vi "FPGAmain_5782_AM_PID.vi"() -> ()   [LabVIEW 2013]
uses:
  FPGA/DataMode.ctl
  FPGA/Input_5782/5782_states.ctl
  <vilib>/Platform/TimedLoop/XDataNode/timing_clust.ctl
  <vilib>/Platform/TimedLoop/XDataNode/nitl_modes.ctl
  <vilib>/Platform/TimedLoop/XDataNode/wakeup.ctl
  <vilib>/rvi/Emulation/niFpgaSctlEmulationGetInTimedLoop.vi
  <vilib>/rvi/Emulation/niFpgaEmulationReportErrorSimple.vi
  <vilib>/rvi/Emulation/niFpgaGetClockAttributes.vi
  <vilib>/rvi/eio/common/nirviEmuTemplateMethod_errors.vi
  <vilib>/rvi/Emulation/niFpgaCriticalErrorInLSC.vi
  <vilib>/rvi/DataTransferAndStorage/Register/Emulation/niFpgaRegisterEmulationFpgaImpl.vi
  <instcachedir>/0/niFpgaRegisterEmulationFpgaImpl_DCF4BC0110594B98B44A971D60CEEC4D.lvgen/niFpgaRegisterEmulationFpgaImpl_DCF4BC0110594B98B44A971D60CEEC4D_003.vi
  <vilib>/rvi/DataTransferAndStorage/Container/Common/niFpgaContainerGetUniqueNameForEmu.vi
  <instcachedir>/0/niFpgaRegisterEmulationFpgaImpl_DCF4BC0110594B98B44A971D60CEEC4D.lvgen/niFpgaRegisterEmulationFpgaImpl_DCF4BC0110594B98B44A971D60CEEC4D_021.vi
  <instcachedir>/0/niFpgaRegisterEmulationFpgaImpl_DCF4BC0110594B98B44A971D60CEEC4D.lvgen/niFpgaRegisterEmulationFpgaImpl_DCF4BC0110594B98B44A971D60CEEC4D_020.vi
  <instcachedir>/0/niFpgaRegisterEmulationFpgaImpl_DCF4BC0110594B98B44A971D60CEEC4D.lvgen/niFpgaRegisterEmulationFpgaImpl_DCF4BC0110594B98B44A971D60CEEC4D_010.vi
  <instcachedir>/0/niFpgaRegisterEmulationFpgaImpl_DCF4BC0110594B98B44A971D60CEEC4D.lvgen/niFpgaRegisterEmulationFpgaImpl_DCF4BC0110594B98B44A971D60CEEC4D_009.vi
  <vilib>/rvi/FIFO/Fifo_Resource/nirvififoEmulationReadFpgaImpl.vi
  <vilib>/rvi/interface/RandomDataEmulation/nirviRandomDataMultiElementFPGAFIFO.vi
  <instcachedir>/0/nirviRandomDataMultiElementFPGAFIFO_F2B80EDE0D7944A08478D8D26097D4DB.lvgen/nirviRandomDataMultiElementFPGAFIFO_F2B80EDE0D7944A08478D8D26097D4DB_005.vi
  <vilib>/rvi/interface/RandomDataEmulation/niFpgaRandomDataHandleErrors.vi
  <instcachedir>/0/niFpgaRegisterEmulationFpgaImpl_DCF4BC0110594B98B44A971D60CEEC4D.lvgen/niFpgaRegisterEmulationFpgaImpl_DCF4BC0110594B98B44A971D60CEEC4D_013.vi
  <vilib>/rvi/interface/RandomDataEmulation/nirviRandomDataFPGAFIFO.vi
  <vilib>/rvi/FIFO/Fifo_Resource/nirvififoEmulationWriteFpgaImpl.vi
  <vilib>/Platform/TimedLoop/XDataNode/XDataNode.xnode
  <vilib>/eio/EIONode/EIONode.xnode
  <vilib>/rvi/DataTransferAndStorage/Container/XNode/niFpgaContainer.xnode
  <vilib>/rvi/DataTransferAndStorage/Register/Emulation/niFpgaRegisterEmulation.vi
  <vilib>/rvi/FIFO/Fifo_Resource/nirvififoEmulationRead.vi
  <vilib>/rvi/interface/RandomDataEmulation/nirviRandomDataFpgaMultiElementTemplate.vi
  <vilib>/rvi/interface/RandomDataEmulation/nirviRandomDataFpgaReadWriteTemplate.vi
  <vilib>/rvi/FIFO/Fifo_Resource/nirvififoEmulationWrite.vi
  <vilib>/Platform/TimedLoop/XDataNode/XDNodeRunTimeDep.lvlib
panel:
  in  "IO Module\\AO Data Sync":bool=TRUE
  in  "IO Module\\SPI Write Data":u16
  out "IO Module\\SPI Read Data":u8
  in  "IO Module\\SPI Read":bool
  in  "IO Module\\SPI Write":bool
  in  "IO Module\\SPI Address":u16
  in  "IO Module\\SPI Device":u8
  out "IO Module\\SPI Idle":bool
  in  "AM phase":fxp<+,64,64>
  in  "delay phase":fxp<+,64,64>
  in  "User Command Commit":bool
  in  "User Command":u8
  out "User Command Idle":bool
  out "User Command Status":u8
  in  "User Data 0":u8
  in  "User Data 1":u8
  out "PLL Locked":bool
  out "User Error":bool
  out "Configured?":bool
  in  "Continuous":bool
  in  "5782 record length":u16=4000 caption="Samples Per Trigger" min=1 step=1
  in  "Trigger Acquisition":bool
  out "IO Module\\Trigger Input":bool
  in  "Downsample":fxp<+,8,8>=1.0
  in  "new coeffs":bool
  in  "FIR coeffs":fxp<+/-,18,18>[](array[numeric])
  in  "CIC Gain":fxp<+/-,32,1>=0.00390625 format="%#_32g"
  in  "Acquisition running":bool
  in  "Phase output":fxp<+,64,64>[](array[numeric])=[0.0, 0.0, 0.0, 0.0, 0.0, 0.0, 0.0, 0.0]
  in  "Simulated phase 5782":fxp<+,64,64>[](array[numeric])=[0.0, 0.0]
  in  "Mode":T1
  in  "Phase 5782":fxp<+,64,64>[](array[numeric])=[0.0, 0.0]
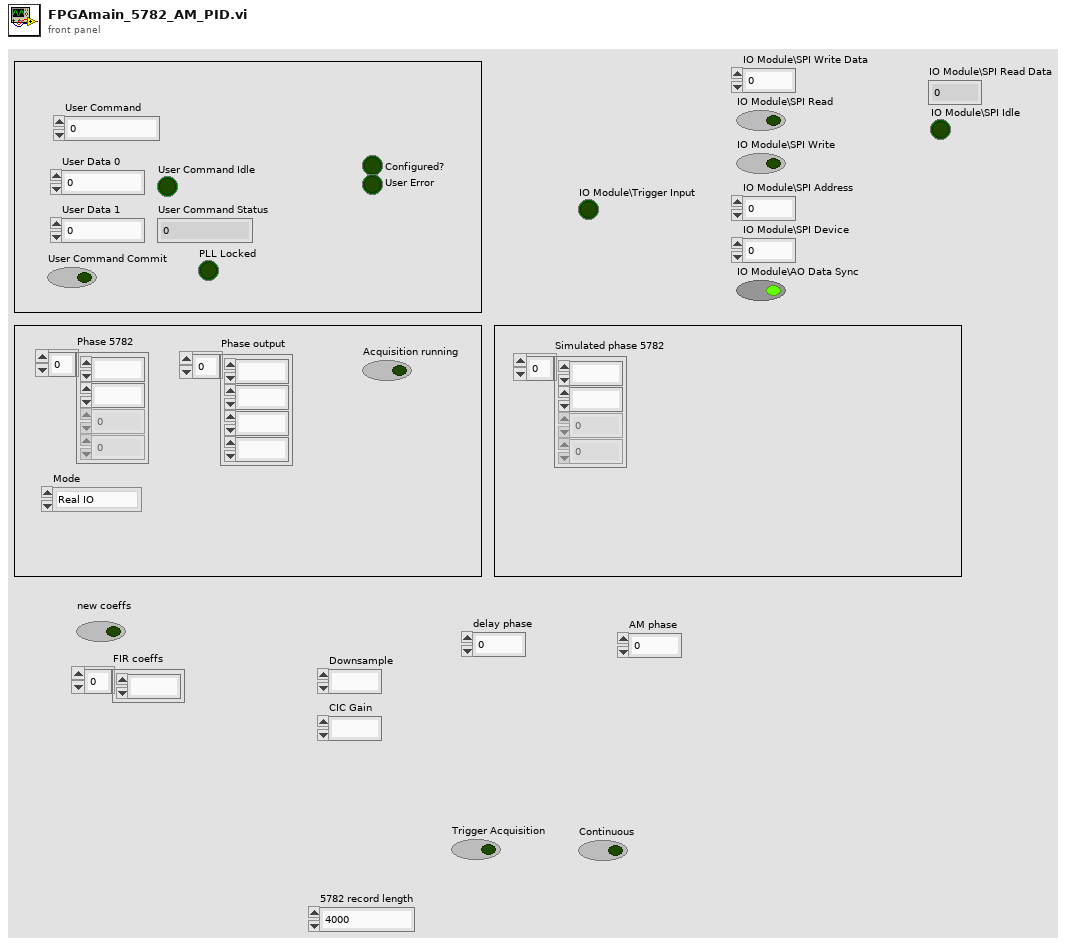
[diagram p1: front panel]
types:
  T1 = typedef "DataMode.ctl" = enum16{"Real IO", "Simulated"}
  T2 = typedef "5782_states.ctl" = enum8{"Wait for trigger", "Acquisition", "Send record length", "Quiet period"}
  T3 = typedef "XDNodeRunTimeDep.lvlib/timing_clust.ctl" = cluster{"Expected End [f-1]":u64, "Actual End [f-1]":u64, "Finished Late? [f-1]":bool, "Expected End [i-1]":u64, "Actual End [i-1]":u64, "Finished Late? [i-1]":bool, "Expected Start [i]":u64, "Actual Start [i]":u64, "Expected Start [f]":u64, "Actual Start [f]":u64, "Source Name":string, "Structure Name":string, "Period":i64, "Deadline":i64, "Offset":i64, "Start":i64, "Priority":i32, "Timeout":i32, "Mode":T4, "Wakeup Reason":T5, "Error":errorcluster, "Source Type":string, "Secondary Source Type":string, "Global End Time":u64, "Global Start Time":u64, "Frame Duration":u64, "Iteration Duration":u64, "Assigned CPU":i32, "I/O Scan Engine Mode":u32}
  T4 = typedef "XDNodeRunTimeDep.lvlib/nitl_modes.ctl" = enum32{"No Change", "Process missed periods, maintain original phase", "Discard missed periods, maintain original phase", "Process missed periods, ignore original phase", "Discard missed periods, ignore original phase"}
  T5 = typedef "XDNodeRunTimeDep.lvlib/wakeup.ctl" = enum32{"Normal", "Aborted", "Asynchronous wakeup", "Timing source error", "Timed loop error", "Timeout"}
  T6 = typedef "I16 array size 2.ctl" = i16[]
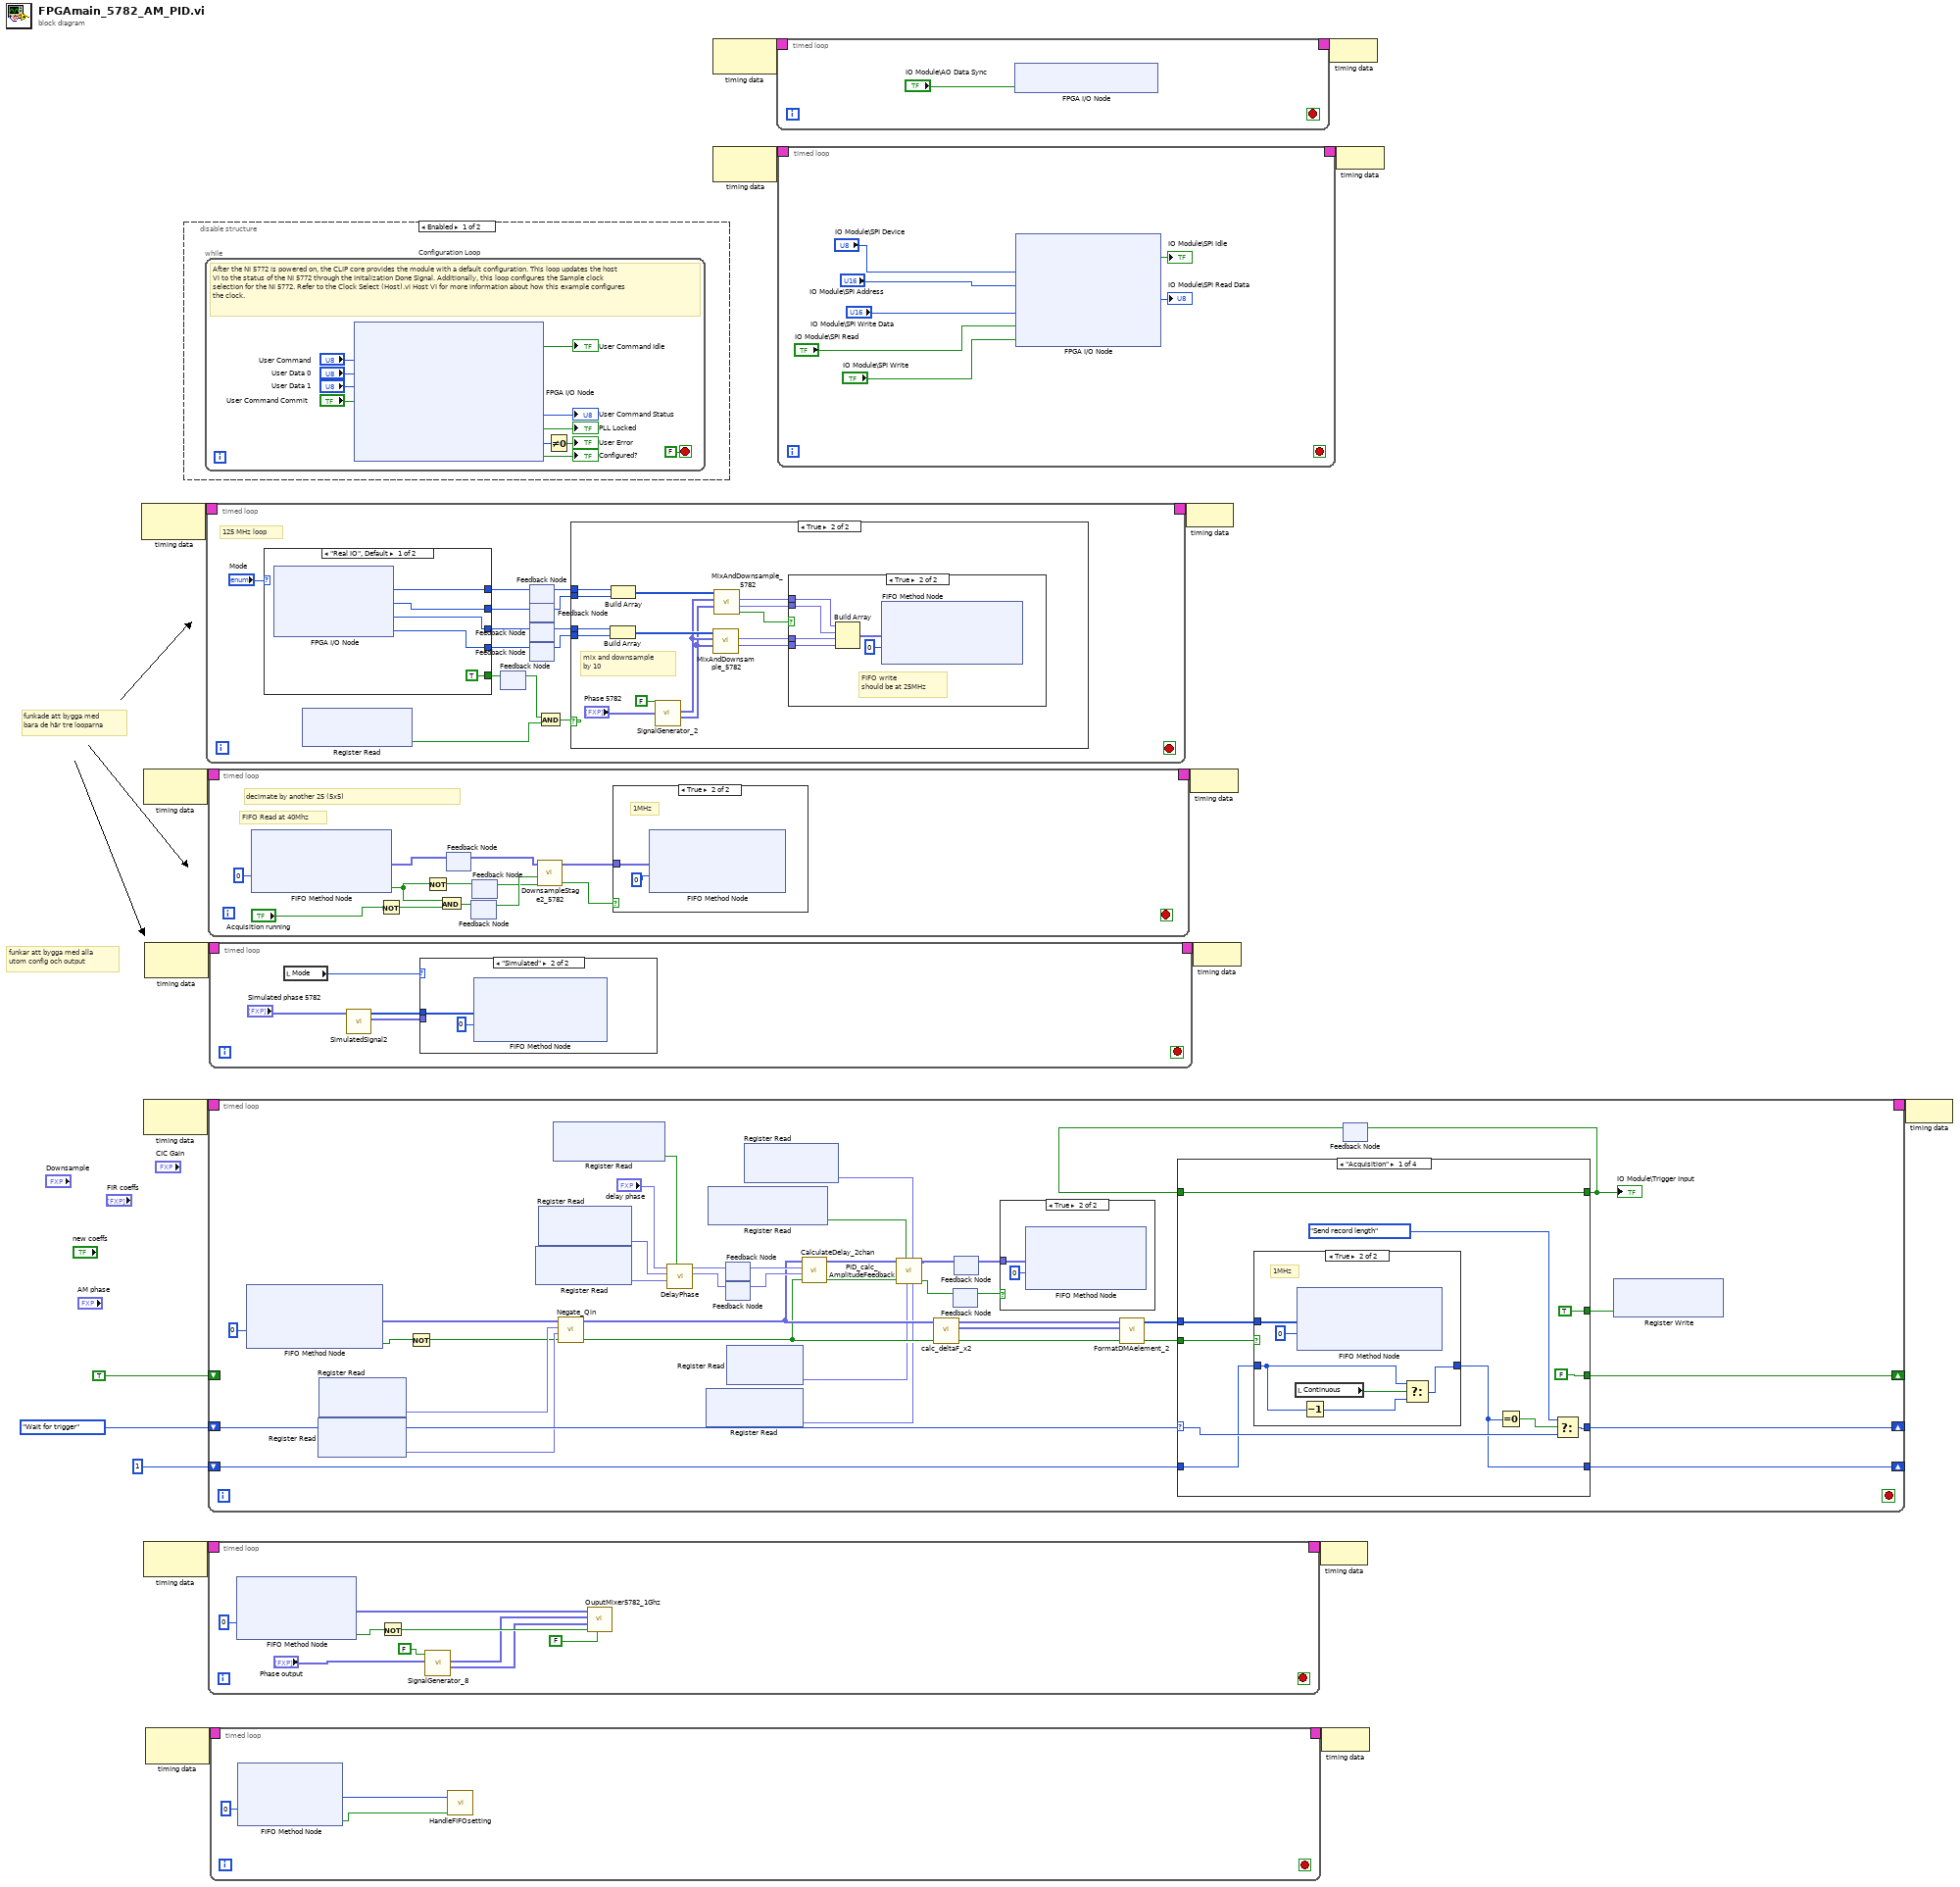
[diagram p0: block diagram]
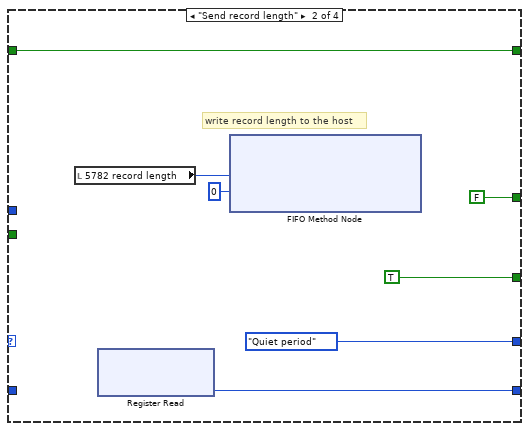
[diagram p4: hidden frame]
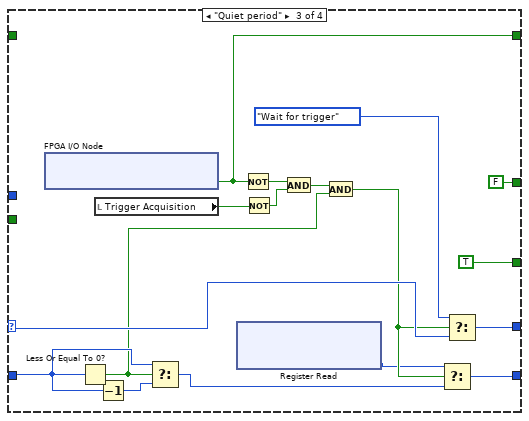
[diagram p5: hidden frame]
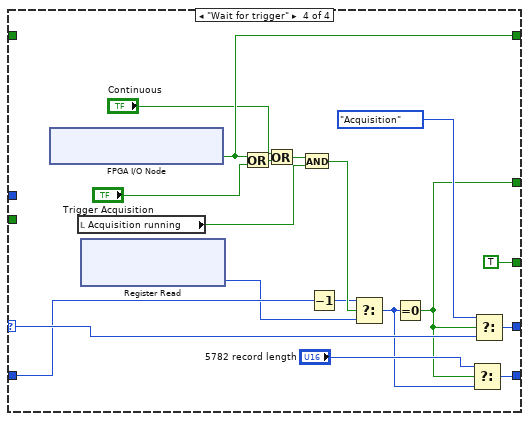
[diagram p6: hidden frame]
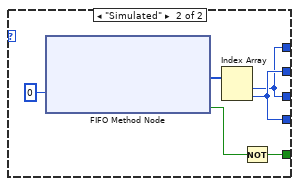
[diagram p10: hidden frame]
diagram:
  # "funkar att bygga med alla\nutom config och output"
  # "funkade att bygga med\nbara de här tre looparna"
  n1 = node-c288() -> (w15:T3)  [unwired: 1 in]
  n2 = node-c288() -> (w19:T3)  [unwired: 1 in]
  n3 = node-c288() -> (w13:T3)  [unwired: 1 in]
  n4 = node-c288() -> (w6:T3)  [unwired: 1 in]
  n5 = node-c288() -> (w17:T3)  [unwired: 1 in]
  n6 = node-c288() -> (w8:T3)  [unwired: 1 in]
  n7 = disable-structure shown="Enabled" {
    frame Enabled {
      n8 = while "Configuration Loop" {
        stop <- FALSE stop-if-true
        # "After the NI 5772 is powered on, the CLIP core provides the module with a default configuration. This loop updates the host VI to the status of the NI 5772 through the Initalization Done Signal. Additionally, this loop configures the Sample clock selection for the NI 5772. Refer to the Clock Select (Host).vi Host VI for more information about how this example configures the clock."
        n9 = xnode "FPGA I/O Node"("IO Module\\User Command"="User Command", "IO Module\\User Data 0"="User Data 0", "IO Module\\User Data 1"="User Data 1", "IO Module\\User Command Commit"="User Command Commit") -> ("IO Module\\User Command Idle"=→"User Command Idle":bool, "IO Module\\User Command Status"=→"User Command Status":u8, "IO Module\\PLL Locked"=→"PLL Locked":bool, "IO Module\\User Error"=w25:u8, "IO Module\\Initialization Done"=→"Configured?":bool)  [unwired: 9 in, 9 out]
        n10 = Not Equal To 0?(x=w25) -> (x != 0?=→"User Error":bool)
      }
    }
    frame Disabled {
    }
  }
  n11 = timed-loop {
    timing: w15 -> [_]
    timing-out: [_] -> w14
    stop <- _ stop-if-true
    # "125 MHz loop"
    n12 = case shown="\"Real IO\", Default" "Mode" {
      tunnel: [w69 w72] -> w41
      tunnel: [w68 w73] -> w39
      tunnel: [w67 w72] -> w37
      tunnel: [w66 w73] -> w34
      tunnel: [TRUE w70] -> w33
      frame "Real IO", Default {
        n13 = xnode "FPGA I/O Node"() -> ("IO Module\\AI 0 N-1"=w69:i16, "IO Module\\AI 0 N"=w68:i16, "IO Module\\AI 1 N-1"=w67:i16, "IO Module\\AI 1 N"=w66:i16)  [unwired: 4 in, 4 out]
      }
      frame "Simulated" {
        n14 = xnode ("FIFO Method Node")("Timeout"=0) -> ("Element"=w74:i16[], "Timed Out?"=w71:bool)  [unwired: 1 in, 1 out]
        n15 = Index Array(array=w74) -> (element #1=w72:i16, element #2=w73:i16)  [unwired: 2 in]
        n16 = Not(x=w71) -> (.not. x?=w70:bool)
      }
    }
    n17 = xnode ("Register Read")() -> ("Data"=w31:bool)  [unwired: 1 in, 1 out]
    n18 = feedback #1() -> (w32:bool)  [unwired: 1 in]
    n19 = feedback-in #1(w33) -> ()
    n20 = feedback #2() -> (w40:i16)  [unwired: 1 in]
    n21 = feedback-in #2(w41) -> ()
    n22 = feedback #3() -> (w38:i16)  [unwired: 1 in]
    n23 = feedback-in #3(w39) -> ()
    n24 = feedback #4() -> (w36:i16)  [unwired: 1 in]
    n25 = feedback-in #4(w37) -> ()
    n26 = feedback #5() -> (w35:i16)  [unwired: 1 in]
    n27 = feedback-in #5(w34) -> ()
    n28 = And(x=w32, y=w31) -> (x .and. y?=w42:bool)
    n29 = case shown="True" w42 {
      tunnel: w40 -> [_ w49]
      tunnel: w38 -> [_ w48]
      tunnel: w36 -> [_ w47]
      tunnel: w35 -> [_ w46]
      frame False {
      }
      frame True {
        # "mix and downsample\nby 10"
        n30 = Build Array(w47, w46) -> (w58:i16[])
        n31 = Build Array(w49, w48) -> (w45:i16[])
        n32 = call "SignalGenerator_2.vi"("Phase"="Phase 5782", "reset"=FALSE) -> ("Sine out"=w50:fxp<+/-,16,0>[], "Cosine out"=w51:fxp<+/-,16,0>[])  [unwired: 8 in]
        n33 = call "MixAndDownsample_5782.vi"("Sine in"=w50, "Cosine in"=w51, "Signal Input"=w58) -> ("Q out"=w53:fxp<+/-,16,14>, "I out"=w54:fxp<+/-,16,14>)  [unwired: 6 in, 1 out]
        n34 = call "MixAndDownsample_5782.vi"("Sine in"=w50, "Cosine in"=w51, "Signal Input"=w45) -> ("data valid"=w55:bool, "Q out"=w56:fxp<+/-,16,14>, "I out"=w57:fxp<+/-,16,14>)  [unwired: 6 in]
        n35 = case shown="True" w55 {
          tunnel: w56 -> [_ w64]
          tunnel: w57 -> [_ w61]
          tunnel: w54 -> [_ w60]
          tunnel: w53 -> [_ w59]
          frame False {
          }
          frame True {
            # "FIFO write\nshould be at 25MHz"
            n36 = Build Array(w61, w64, w60, w59) -> (w63:fxp<+/-,16,14>[])
            n37 = xnode ("FIFO Method Node")("Element"=w63, "Timeout"=0) -> ()  [unwired: 1 in, 2 out]
          }
        }
      }
    }
  }
  n38 = timed-loop {
    timing: w19 -> [_]
    timing-out: [_] -> w18
    stop <- _ stop-if-true
    # "FIFO Read at 40Mhz"
    # "decimate by another 25 (5x5)"
    n39 = xnode ("FIFO Method Node")("Timeout"=0) -> ("Element"=w83:fxp<+/-,16,14>[], "Timed Out?"=w85:bool)  [unwired: 1 in, 1 out]
    n40 = Not(x="Acquisition running") -> (.not. x?=w86:bool)
    n41 = Not(x=w85) -> (.not. x?=w79:bool)
    n42 = And(x=w85, y=w86) -> (x .and. y?=w81:bool)
    n43 = feedback #6() -> (w82:fxp<+/-,16,14>[])  [unwired: 1 in]
    n44 = feedback-in #6(w83) -> ()
    n45 = feedback #7() -> (w80:bool)  [unwired: 1 in]
    n46 = feedback-in #7(w81) -> ()
    n47 = feedback #8() -> (w78:bool)  [unwired: 1 in]
    n48 = feedback-in #8(w79) -> ()
    n49 = call "DownsampleStage2_5782.vi"("valid in"=w78, "reset"=w80, "Data in"=w82) -> ("valid out"=w87:bool, "data out"=w88:fxp<+/-,16,14>[])  [unwired: 7 in]
    n50 = case shown="True" w87 {
      tunnel: w88 -> [_ w90]
      frame False {
      }
      frame True {
        # "1MHz"
        n51 = xnode ("FIFO Method Node")("Element"=w90, "Timeout"=0) -> ()  [unwired: 1 in, 2 out]
      }
    }
  }
  n52 = timed-loop {
    timing: w13 -> [_]
    timing-out: [_] -> w12
    shift-right: [w130] -> _
    shift-left: 5782_states."Wait for trigger" ("5782 states") -> [w132]
    shift-right: [w129] -> _
    shift-left: u16 1 ("trigger samples") -> [w131]
    shift-right: [w124] -> _
    shift-left: TRUE -> [_]
    stop <- _ stop-if-true
    n53 = xnode ("FIFO Method Node")("Timeout"=0) -> ("Element"=w98:fxp<+/-,16,14>[], "Timed Out?"=w127:bool)  [unwired: 1 in, 1 out]
    n54 = xnode ("Register Read")() -> ("Data"=w109:fxp<+/-,16,14>)  [unwired: 1 in, 1 out]
    n55 = xnode ("Register Read")() -> ("Data"=w110:fxp<+/-,16,14>)  [unwired: 1 in, 1 out]
    n56 = Not(x=w127) -> (.not. x?=w99:bool)
    n57 = xnode ("Register Read")() -> ("Data"=w106:fxp<+/-,16,0>)  [unwired: 1 in, 1 out]
    n58 = xnode ("Register Read")() -> ("Data"=w107:fxp<+/-,16,0>)  [unwired: 1 in, 1 out]
    n59 = xnode ("Register Read")() -> ("Data"=w108:bool)  [unwired: 1 in, 1 out]
    n60 = call "Negate_Qin.vi"("valid in"=w99, "DC offset chan 1"=w109, "DC offset chan 0"=w110, "Data in"=w98) -> ("valid out"=w113:bool, "Data out"=w118:fxp<+/-,16,14>[])  [unwired: 6 in]
    n61 = call "DelayPhase.vi"("Use fixed delay"=w108, "fixed cos_fi"=w106, "fixed sin fi"=w107, "delay phase"="delay phase") -> ("cos_fi"=w115:fxp<+/-,16,0>, "sin fi"=w116:fxp<+/-,16,0>)  [unwired: 6 in]
    n62 = xnode ("Register Read")() -> ("Data"=w101:fxp<+/-,32,6>)  [unwired: 1 in, 1 out]
    n63 = xnode ("Register Read")() -> ("Data"=w103:bool)  [unwired: 1 in, 1 out]
    n64 = feedback-in #9(w116) -> ()
    n65 = feedback #9() -> (w120:fxp<+/-,16,0>)  [unwired: 1 in]
    n66 = feedback #10() -> (w119:fxp<+/-,16,0>)  [unwired: 1 in]
    n67 = feedback-in #10(w115) -> ()
    n68 = xnode ("Register Read")() -> ("Data"=w102:fxp<+/-,32,6>)  [unwired: 1 in, 1 out]
    n69 = xnode ("Register Read")() -> ("Data"=w100:fxp<+/-,32,6>)  [unwired: 1 in, 1 out]
    n70 = call "CalculateDelay_2chan.vi"("input valid"=w113, "cos_fi"=w119, "sin fi"=w120, "Data in"=w118) -> ("output valid"=w104:bool, "Data out"=w105:fxp<+/-,16,14>[])  [unwired: 6 in]
    n71 = call "PID_calc_AmplitudeFeedback.vi"("Kd/Tau"=w101, "Ki*Tau"=w100, "Kp"=w102, "Enabled"=w103, "input valid"=w104, "Data in"=w105) -> ("output valid"=w95:bool, "data out"=w97:fxp<+/-,16,14>[])  [unwired: 2 in, 2 out]
    n72 = call "calc_deltaF_x2.vi"("valid in"=w113, "Data in"=w118) -> ("valid out"=w112:bool, "deltaF"=w111:fxp<+/-,32,30>[], "Data out"=w114:fxp<+/-,16,14>[])  [unwired: 7 in]
    n73 = feedback #11() -> (w94:bool)  [unwired: 1 in]
    n74 = feedback-in #11(w95) -> ()
    n75 = feedback #12() -> (w96:fxp<+/-,16,14>[])  [unwired: 1 in]
    n76 = feedback-in #12(w97) -> ()
    n77 = case shown="True" w94 {
      tunnel: w96 -> [_ w133]
      frame False {
      }
      frame True {
        n78 = xnode ("FIFO Method Node")("Element"=w133, "Timeout"=0) -> ()  [unwired: 1 in, 2 out]
      }
    }
    n79 = call "FormatDMAelement_2.vi"("valid in"=w112, "deltaF"=w111, "Data in"=w114) -> ("valid out"=w125:bool, "Element"=w126:u64[])  [unwired: 7 in]
    n80 = feedback #13() -> (w122:bool)  [unwired: 1 in]
    n81 = case shown="\"Acquisition\"" w132 {
      selector: w132 -> [w145 _ w175 w194]
      tunnel: w131 -> [w141 _ w163 w181]
      tunnel: [w144 5782_states."Quiet period" ("5782 states") w174 w193] -> w130
      tunnel: [w138 w153 w176 w192] -> w129
      tunnel: w126 -> [w139 _ _ _]
      tunnel: w125 -> [w140 _ _ _]
      tunnel: [FALSE TRUE TRUE TRUE] -> w124
      tunnel: [TRUE FALSE ("5782 triggered") FALSE ("5782 triggered") w185] -> w123
      tunnel: [w137 w154 w165 w184] -> w121
      tunnel: w122 -> [w137 w154 _ _]
      frame "Acquisition" {
        n82 = case shown="True" w140 {
          tunnel: w139 -> [_ w152]
          tunnel: [w146 w149] -> w138
          tunnel: w141 -> [w146 w147]
          frame False {
          }
          frame True {
            # "1MHz"
            n83 = local read "Continuous"() -> (w150:bool)
            n84 = xnode ("FIFO Method Node")("Element"=w152, "Timeout"=0) -> ()  [unwired: 1 in, 2 out]
            n85 = Decrement(x=w147) -> (x-1=w148:u16)
            n86 = Select(t=w147, s=w150, f=w148) -> (s? t:f=w149:u16)
          }
        }
        n87 = Equal To 0?(x=w138) -> (x = 0?=w142:bool)
        n88 = Select(t=5782_states."Send record length" ("5782 states"), s=w142, f=w145) -> (s? t:f=w144:T2)
      }
      frame "Send record length" {
        # "write record length to the host"
        n89 = local read "5782 record length"() -> (w156:u16)
        n90 = xnode ("Register Read")() -> ("Data"=w153:u16)  [unwired: 1 in, 1 out]
        n91 = xnode ("FIFO Method Node")("Element"=w156, "Timeout"=0) -> ()  [unwired: 1 in, 2 out]
      }
      frame "Quiet period" {
        n92 = xnode "FPGA I/O Node"() -> ("IO Module\\Trigger Input"=w165:bool)  [unwired: 1 in, 1 out]
        n93 = Less Or Equal To 0?(x=w163) -> (x <= 0?=w162:bool)
        n94 = local read "Trigger Acquisition"() -> (w171:bool)
        n95 = Decrement(x=w163) -> (x-1=w164:u16)
        n96 = Select(t=w163, s=w162, f=w164) -> (s? t:f=w161:u16)
        n97 = xnode ("Register Read")() -> ("Data"=w160:u16)  [unwired: 1 in, 1 out]
        n98 = Not(x=w165) -> (.not. x?=w170:bool)
        n99 = Not(x=w171) -> (.not. x?=w169:bool)
        n100 = And(x=w170, y=w169) -> (x .and. y?=w168:bool)
        n101 = And(x=w168, y=w162) -> (x .and. y?=w173:bool)
        n102 = Select(t=w160, s=w173, f=w161) -> (s? t:f=w176:u16)
        n103 = Select(t=5782_states."Wait for trigger" ("5782 states"), s=w173, f=w175) -> (s? t:f=w174:T2)
      }
      frame "Wait for trigger" {
        n104 = xnode "FPGA I/O Node"() -> ("IO Module\\Trigger Input"=w184:bool)  [unwired: 1 in, 1 out]
        n105 = local read "Acquisition running"() -> (w186:bool)
        n106 = xnode ("Register Read")() -> ("Data"=w177:u16)  [unwired: 1 in, 1 out]
        n107 = Or(x=w184, y="Trigger Acquisition") -> (x .or. y?=w180:bool)
        n108 = Or(x="Continuous", y=w180) -> (x .or. y?=w178:bool)
        n109 = And(x=w178, y=w186) -> (x .and. y?=w187:bool)
        n110 = Decrement(x=w181) -> (x-1=w182:u16)
        n111 = Select(t=w182, s=w187, f=w177) -> (s? t:f=w183:u16)
        n112 = Equal To 0?(x=w183) -> (x = 0?=w185:bool)
        n113 = Select(t="5782 record length", s=w185, f=w183) -> (s? t:f=w192:u16)
        n114 = Select(t=5782_states."Acquisition" ("5782 states"), s=w185, f=w194) -> (s? t:f=w193:T2)
      }
    }
    "IO Module\\Trigger Input" <- w121
    n115 = feedback-in #13(w121) -> ()
    n116 = xnode ("Register Write")("Data"=w123) -> ()  [unwired: 1 in, 1 out]
  }
  n117 = timed-loop {
    timing: w6 -> [_]
    timing-out: [_] -> w5
    stop <- _ stop-if-true
    n118 = xnode ("FIFO Method Node")("Timeout"=0) -> ("Element"=w201:fxp<+/-,16,14>[], "Timed Out?"=w204:bool)  [unwired: 1 in, 1 out]
    n119 = Not(x=w204) -> (.not. x?=w200:bool)
    n120 = call "SignalGenerator_8.vi"("Phase"="Phase output", "reset"=FALSE) -> ("Sine out"=w197:fxp<+/-,16,0>[], "Cosine out"=w198:fxp<+/-,16,0>[])  [unwired: 8 in]
    n121 = call "OuputMixer5782_1Ghz.vi"("reset"=FALSE, "valid in"=w200, "Sine in"=w197, "Cosine in"=w198, "Data in"=w201) -> ()  [unwired: 5 in, 2 out]
  }
  n122 = timed-loop {
    timing: w17 -> [_]
    timing-out: [_] -> w16
    stop <- _ stop-if-true
    n123 = local read "Mode"() -> (w211:T1)
    n124 = call "SimulatedSignal2.vi"("Phase"="Simulated phase 5782") -> ("dummy do not use"=w208:fxp<+/-,16,0>[], "output"=w210:T6)  [unwired: 9 in]
    n125 = case shown="\"Simulated\"" w211 {
      tunnel: w210 -> [_ w212]
      tunnel: w208 -> [_ _]
      frame "Real IO", Default {
      }
      frame "Simulated" {
        n126 = xnode ("FIFO Method Node")("Element"=w212, "Timeout"=0) -> ()  [unwired: 1 in, 2 out]
      }
    }
  }
  n127 = timed-loop {
    timing: w8 -> [_]
    timing-out: [_] -> w7
    stop <- _ stop-if-true
    n128 = xnode ("FIFO Method Node")("Timeout"=0) -> ("Element"=w217:u64, "Timed Out?"=w216:bool)  [unwired: 1 in, 1 out]
    n129 = call "HandleFIFOsetting.vi"("timed out"=w216, "Value"=w217) -> ()  [unwired: 10 in]
  }
  n130 = node-c288() -> (w2:T3)  [unwired: 1 in]
  n131 = node-c288() -> (w4:T3)  [unwired: 1 in]
  n132 = timed-loop {
    timing: w2 -> [_]
    timing-out: [_] -> w1
    stop <- _ stop-if-true
    n133 = xnode "FPGA I/O Node"("IO Module\\AO Data Sync"="IO Module\\AO Data Sync") -> ()  [unwired: 1 in, 1 out]
  }
  n134 = timed-loop {
    timing: w4 -> [_]
    timing-out: [_] -> w3
    stop <- _ stop-if-true
    n135 = xnode "FPGA I/O Node"("IO Module\\SPI Device"="IO Module\\SPI Device", "IO Module\\SPI Address"="IO Module\\SPI Address", "IO Module\\SPI Write Data"="IO Module\\SPI Write Data", "IO Module\\SPI Read"="IO Module\\SPI Read", "IO Module\\SPI Write"="IO Module\\SPI Write") -> ("IO Module\\SPI Idle"=→"IO Module\\SPI Idle":bool, "IO Module\\SPI Read Data"=→"IO Module\\SPI Read Data":u8)  [unwired: 7 in, 7 out]
  }
  n136 = node-c288(w14) -> ()
  n137 = node-c288(w18) -> ()
  n138 = node-c288(w16) -> ()
  n139 = node-c288(w5) -> ()
  n140 = node-c288(w7) -> ()
  n141 = node-c288(w1) -> ()
  n142 = node-c288(w3) -> ()
  n143 = node-c288(w12) -> ()
